vi "EmptyClipboard.vi"(4 "error in (no error)":errorcluster) -> (0 "error out":errorcluster)   [LabVIEW 2011]
uses:
  user32.dll
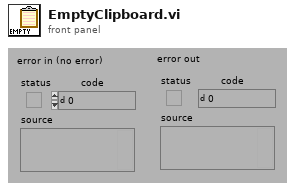
[diagram p1: front panel]
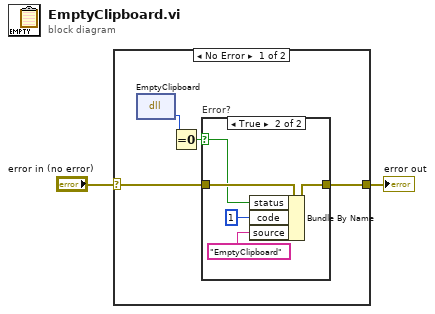
[diagram p0: block diagram]
diagram:
  n1 = case shown="No Error" "error in (no error)" {
    selector: "error in (no error)" -> [w3 w13]
    tunnel: [w4 w13] -> w2
    frame No Error {
      n2 = dll-call lib="User32.dll" fn="EmptyClipboard" label="unsigned long EmptyClipboard(void);"() -> (w6:u32)  [unwired: 3 in, 2 out]
      n3 = Equal To 0?(x=w6) -> (x = 0?=w5:bool)
      n4 = case "Error?" shown="True" w5 {
        selector: w5 -> [_ w11]
        tunnel: w3 -> [w7 w12]
        tunnel: [w7 w8] -> w4
        frame False {
        }
        frame True {
          n5 = Bundle By Name(cluster=w12, "status"=w11, "code"=1, "source"="EmptyClipboard") -> (w8:errorcluster)
        }
      }
    }
    frame Error {
    }
  }
  "error out" <- w2
